vi "Main.vi"() -> ()   [LabVIEW 2021]
doc: "This vi acts as an user interface to display acquire data and save data when required. User can ineract with the panel to choose file (CSV or TDMS) and data display type(chart or graph). It also allow user to select channel index and define channel name, scale and offset. It then can let user choose a moment to start recording either on defined time length or user choice."
uses:
  Control/Data Display Choice Enum.ctl
  Control/File Choice Enum.ctl
  Control/User Interface Reference Cluster.ctl
  Control/Data Display Manager Enum.ctl
  Control/Volt Chl.ctl
  Control/File Manager Enum.ctl
  Control/Command and Data Cluster.ctl
  Control/DAQ Manager Enum.ctl
  <extravilib>/ChannelInstances/Stream-a[.](wfm(dbl))/Read With Abort.vi
  <extravilib>/ChannelInstances/Stream-a[.](wfm(dbl))/Write With Abort.vi
  <extravilib>/ChannelInstances/Stream-a[.](wfm(dbl))/EndpointRead.vi
  <extravilib>/ChannelInstances/Stream-a[.](wfm(dbl))/Endpoint.vi
  <extravilib>/ChannelInstances/Stream-a[.](wfm(dbl))/Instantiate.vi
  <extravilib>/ChannelInstances/Event Messenger-t'Command and Data Cluster.ctl'/Instantiate.vi
  <extravilib>/ChannelInstances/Event Messenger-t'Command and Data Cluster.ctl'/))Channel.vi
  <extravilib>/ChannelInstances/Stream-a[.](wfm(dbl))/)Channel.vi
  <resource>/ChannelSupport/_ChannelSupport/WaitIfNeeded.vi
  <extravilib>/ChannelInstances/Event Messenger-t'Command and Data Cluster.ctl'.lvlib
  <extravilib>/ChannelInstances/Stream-a[.](wfm(dbl)).lvlib
panel:
  out "Error":errorcluster
  out "Overall Raw \nVoltage Mean":dbl[](array[numeric])
  out "Raw Voltage Mean \nper Second":dbl[](array[numeric])
  out "Recording":bool
  in  "File Choice":T1=enum."CSV File"
  in  "DD Choice":T2 caption="Data Display Choice"
  out "File Path":path
  in  "Choice Ok":bool
  in  "File Name":string
  in  "Exit":bool
  in  "Use Re Time":bool caption="Use Record Time"
  in  "Re Time":dbl=10.0 caption="Record Time (s)"
  in  "Device Name":tag
  in  "Sample Rate":i32=100 caption="Sample Rate (S/s)"
  in  "Init Button":bool
  in  "Record":bool
  in  "Start":bool
  in  "Stop":bool
  out "element":waveform(dbl)[](array[waveform])
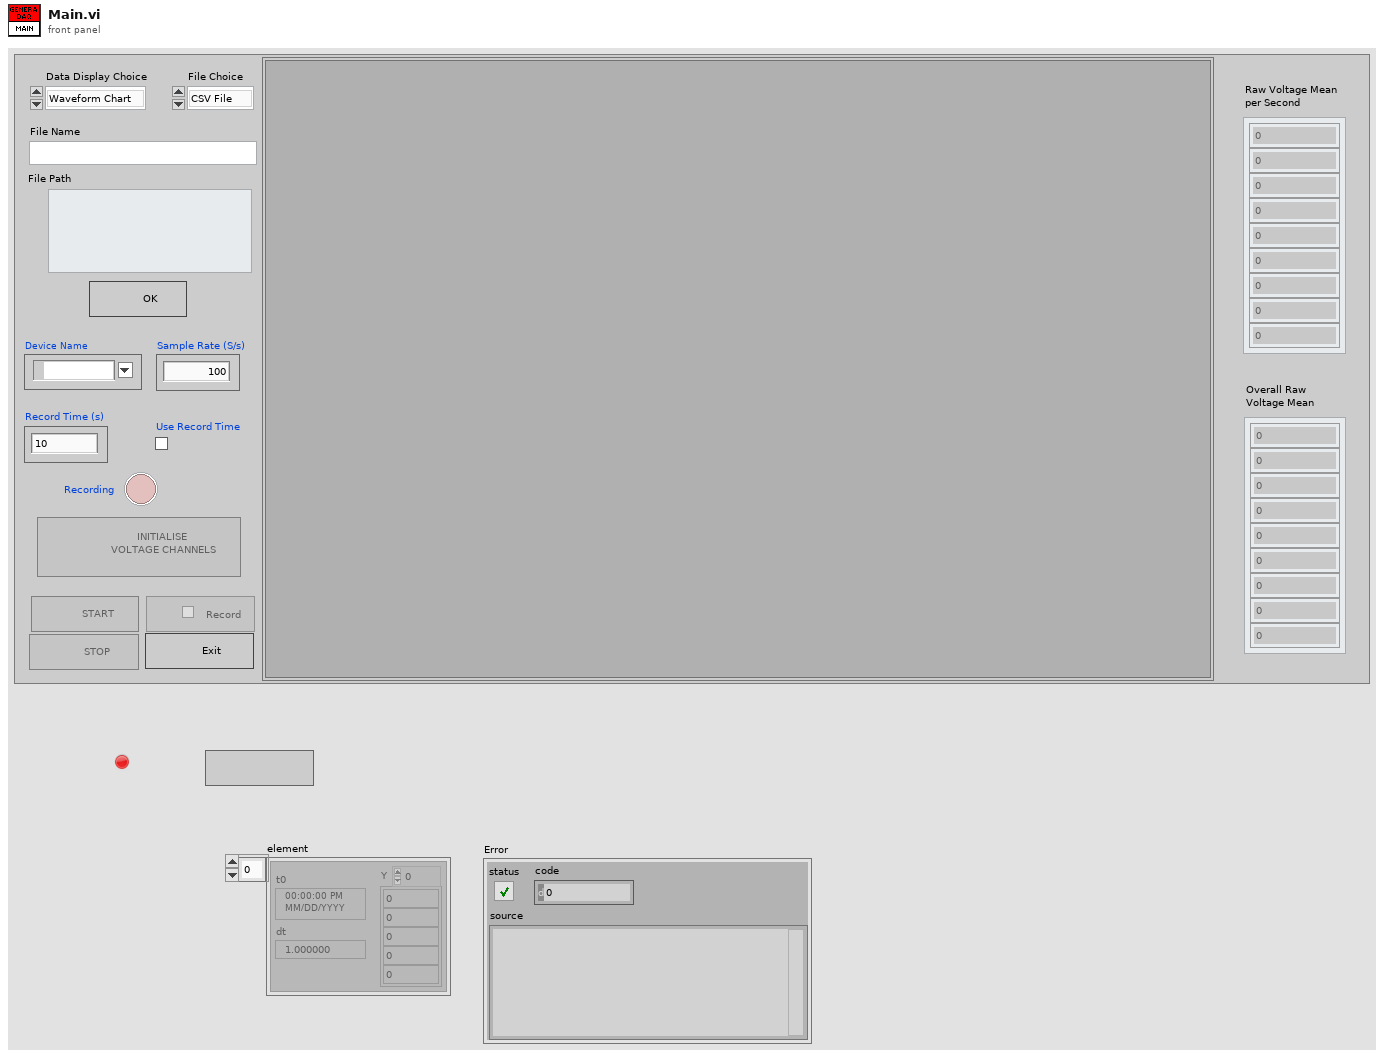
[diagram p1: front panel]
types:
  T1 = typedef "File Choice Enum.ctl" = enum16{"TDMS File", "CSV File"}
  T2 = typedef "Data Display Choice Enum.ctl" = enum16{"Waveform Chart", "Waveform Graph"}
  T3 = typedef "User Interface Reference Cluster.ctl" = cluster{"Choice Ok":refnum<vi>, "Init Button":refnum<vi>, "Start":refnum<vi>, "Record":refnum<vi>, "Stop":refnum<vi>, "Exit":refnum<vi>, "File Choice":refnum<vi>, "DD Choice":refnum<vi>}
  T4 = typedef "Command and Data Cluster.ctl" = cluster{"Command":string, "Data":variant}
  T5 = typedef "Event Messenger-t'Command and Data Cluster.ctl'.lvlib/))Channel.ctl" = refnum<queue>
  T6 = typedef "DAQ Manager Enum.ctl" = enum16{"Config", "Start", "Read", "Stop"}
  T7 = typedef "Volt Chl.ctl" = cluster{"Index":i32[], "Chl Name":string[], "Scale":dbl[], "Offset":dbl[], "Sample Rate":i32, "Device Name":tag, "Channel":tag}
  T8 = typedef "Stream-a[.](wfm(dbl)).lvlib/)Channel.ctl" = refnum<queue>
  T9 = typedef "Data Display Manager Enum.ctl" = enum16{"Display Choice", "Config Data", "Volt Data"}
  T10 = typedef "File Manager Enum.ctl" = enum16{"Create File", "Config Data", "Volt Data", "Set Time", "Close File"}
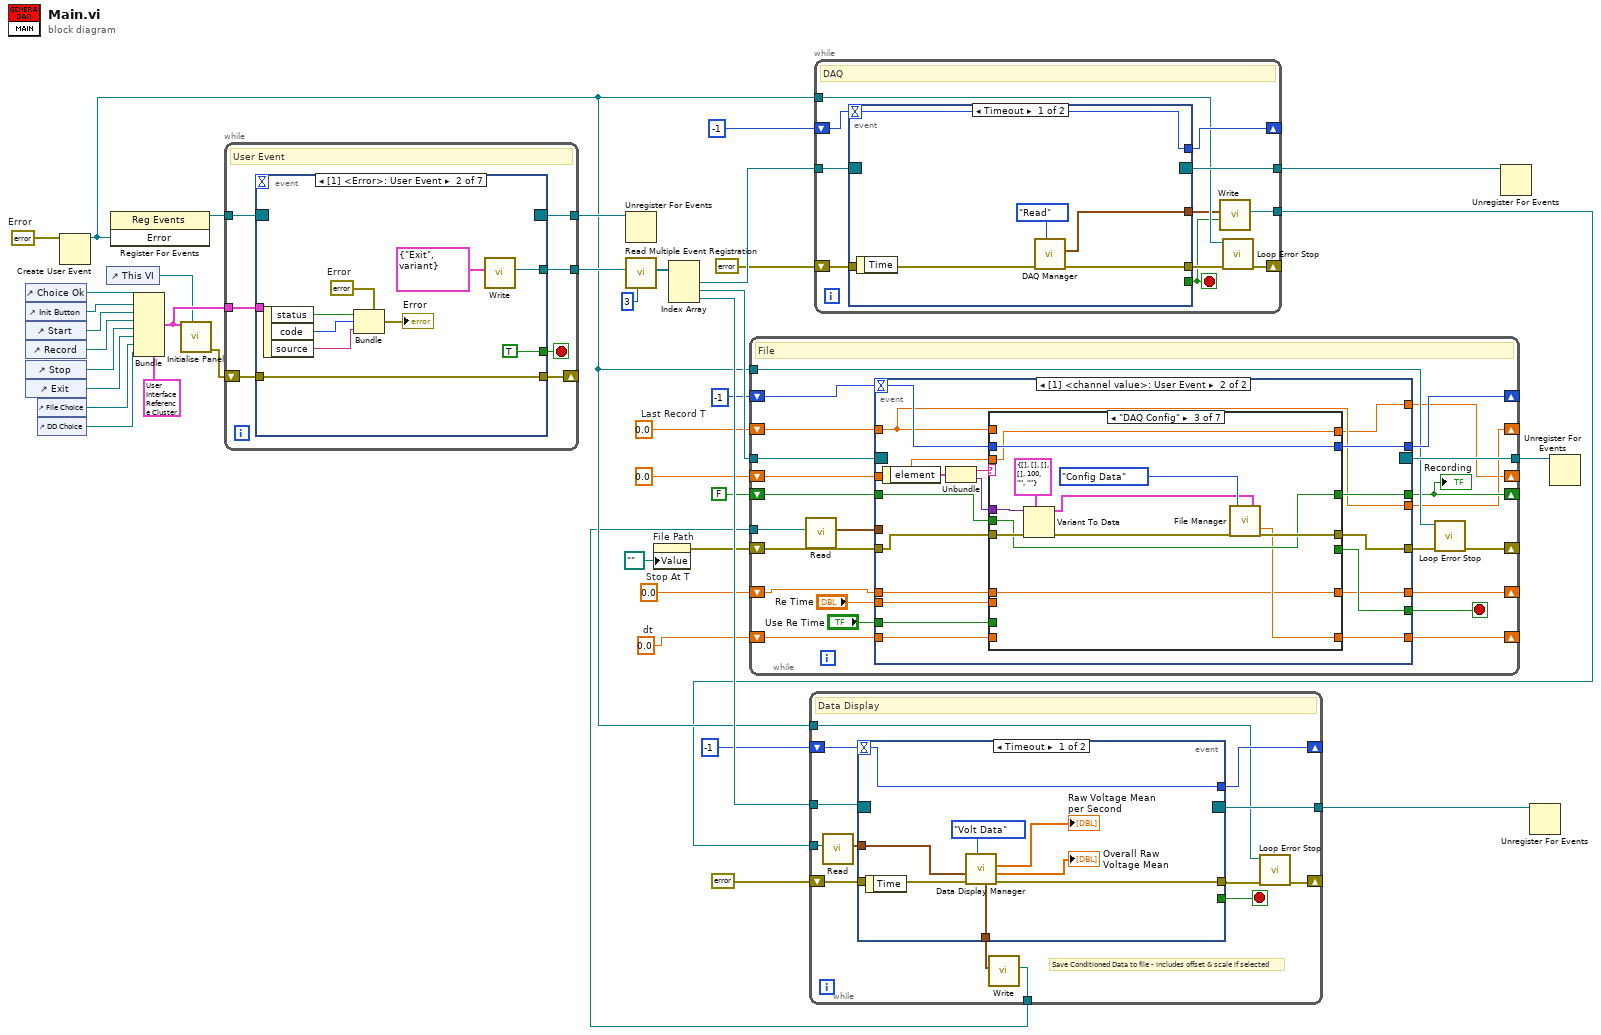
[diagram p0: block diagram]
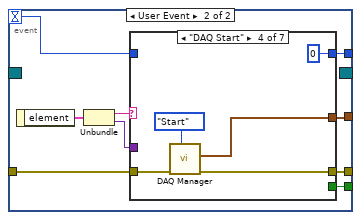
[diagram p2: hidden frame]
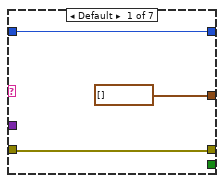
[diagram p3: hidden frame]
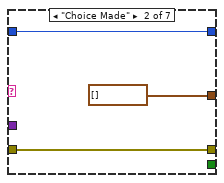
[diagram p4: hidden frame]
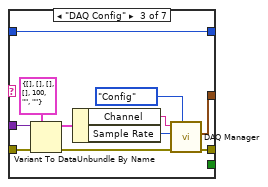
[diagram p5: hidden frame]
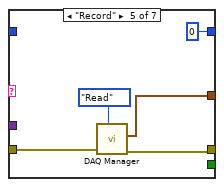
[diagram p6: hidden frame]
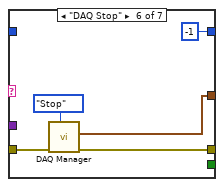
[diagram p7: hidden frame]
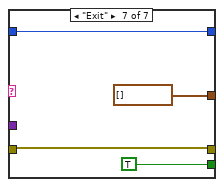
[diagram p8: hidden frame]
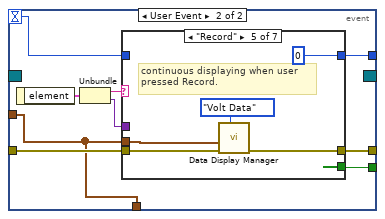
[diagram p9: hidden frame]
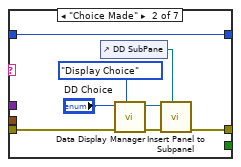
[diagram p11: hidden frame]
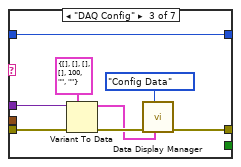
[diagram p12: hidden frame]
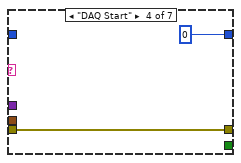
[diagram p13: hidden frame]
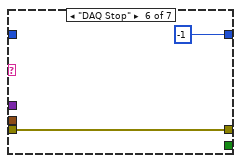
[diagram p14: hidden frame]
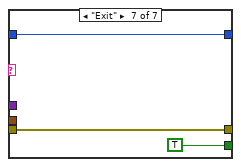
[diagram p15: hidden frame]
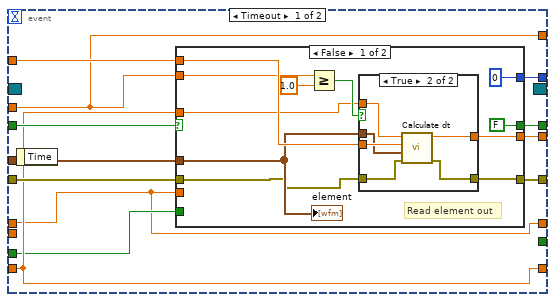
[diagram p16: hidden frame]
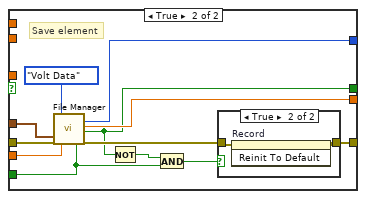
[diagram p18: hidden frame]
diagram:
  w3 = 0.0  # Stop At T
  w5 = 0.0  # dt
  w6 = 0.0  # Last Record T
  w10 = errorcluster {"status"=FALSE, "code"=0, "source"=""}  # Error
  n1 = control-ref of="Choice Ok"() -> (w27:refnum<vi>)
  n2 = control-ref of="Init Button"() -> (w26:refnum<vi>)
  n3 = control-ref of="Start"() -> (w25:refnum<vi>)
  n4 = control-ref of="Record"() -> (w24:refnum<vi>)
  n5 = control-ref of="Stop"() -> (w23:refnum<vi>)
  n6 = control-ref of="Exit"() -> (w22:refnum<vi>)
  n7 = control-ref of="File Choice"() -> (w21:refnum<vi>)
  n8 = control-ref of="DD Choice"() -> (w20:refnum<vi>)
  n9 = Create User Event(user event datatype=w10) -> (user event=w12:refnum<user-event>)  [unwired: 1 in, 1 out]
  n10 = control-ref of="This VI"() -> (w11:refnum<vi>)
  n11 = register-events(w12) -> (reference out=w14:refnum<event-registration>)  [unwired: 2 in, 1 out]
  n12 = Bundle(cluster=T3 {"Choice Ok"=refnum, "Init Button"=refnum, "Start"=refnum, "Record"=refnum, "Stop"=refnum, "Exit"=refnum, "File Choice"=refnum, "DD Choice"=refnum} ("output cluster"), "Choice Ok"=w27, "Init Button"=w26, "Start"=w25, "Record"=w24, "Stop"=w23, "Exit"=w22, "File Choice"=w21, "DD Choice"=w20) -> (w17:T3)
  n13 = call "Initialise Panel.vi"("This VI"=w11, "UI Ref"=w17) -> ("error out"=w18:errorcluster)  [unwired: 9 in]
  n14 = while {
    tunnel: [w45] -> w33
    tunnel: w17 -> [w44]
    tunnel: w14 -> [w43]
    tunnel: [w42] -> w13
    shift-right: [w40] -> _
    shift-left: w18 -> [w41]
    stop <- w46 stop-if-true
    # "User Event"
    n15 = event shown="[1] <Error>: User Event" {
      selector: w43 -> [_ _ _ _ _ _ _]
      dyn-events: [_ _ _ _ _ _ _] -> w42
      timeout: _ -> [_ _ _ _ _ _ _]
      tunnel: [TRUE TRUE _ _ _ _ _] -> w46
      tunnel: [w48 w57 w73 w90 w107 w113 w130] -> w45
      tunnel: w44 -> [_ _ w72 w85 w99 _ w129]
      tunnel: w41 -> [w47 w51 w60 w75 w93 w108 w118]
      tunnel: [w47 w51 w61 w76 w94 w108 w114] -> w40
      event "Exit": Value Change {
        n16 = event-data() -> ()  [unwired: 1 in, 1 out]
        n17 = call <extravilib>:"Write.vi"("element"=T4 {"Command"="Exit", "Data"=variant} ("Cluster")) -> ("channel"=w48:T5)  [unwired: 9 in, 1 out]
      }
      event User Event {
        w56 = errorcluster {"status"=FALSE, "code"=0, "source"=""}  # Error
        n18 = event-data() -> ("status"=w55:bool, "code"=w54:i32, "source"=w53:string)  [unwired: 1 in]
        n19 = Bundle(cluster=w56, "status"=w55, "code"=w54, "source"=w53) -> (→"Error":errorcluster)
        n20 = call <extravilib>:"Write.vi"("element"=T4 {"Command"="Exit", "Data"=variant} ("Cluster")) -> ("channel"=w57:T5)  [unwired: 9 in, 1 out]
      }
      event "Choice Ok": Value Change {
        n21 = event-data() -> ()  [unwired: 1 in, 1 out]
        n22 = Unbundle By Name(w72) -> ("File Choice"=w65:refnum<vi>, "DD Choice"=w64:refnum<vi>, "Choice Ok"=w71:refnum<vi>, "Init Button"=w70:refnum<vi>)
        n23 = Build Array(w65, w64, w71) -> (w68:refnum<vi>[])
        n24 = Build Array(w70) -> (w66:refnum<vi>[])
        n25 = call "Enable UI.vi"("Enable?"=FALSE, "output cluster"=w68) -> ("error out"=w63:errorcluster)  [unwired: 9 in]
        n26 = call "Enable UI.vi"("Enable?"=TRUE, "output cluster"=w66) -> ("error out"=w62:errorcluster)  [unwired: 9 in]
        n27 = call <extravilib>:"Write.vi"("element"=T4 {"Command"="Choice Made", "Data"=variant} ("Cluster")) -> ("channel"=w73:T5)  [unwired: 9 in, 1 out]
        n28 = Merge Errors(w63, w62, w60) -> (w61:errorcluster)
      }
      event "Init Button": Value Change {
        n29 = event-data() -> ()  [unwired: 1 in, 1 out]
        n30 = Unbundle By Name(w85) -> ("Init Button"=w80:refnum<vi>, "Start"=w79:refnum<vi>)
        n31 = Build Array(w80) -> (w84:refnum<vi>[])
        n32 = Build Array(w79) -> (w83:refnum<vi>[])
        n33 = call "DAQ Channel Dlg_V0.vi"("DAQ Sample Rate (S/s)"="Sample Rate", "Device Name"="Device Name") -> ("Chl Infor"=w86:variant)  [unwired: 9 in]
        n34 = call "Enable UI.vi"("Enable?"=FALSE, "output cluster"=w84) -> ("error out"=w77:errorcluster)  [unwired: 9 in]
        n35 = call "Enable UI.vi"("Enable?"=TRUE, "output cluster"=w83) -> ("error out"=w78:errorcluster)  [unwired: 9 in]
        n36 = Bundle(cluster=T4 {"Command"="DAQ Config", "Data"=variant} ("Cluster"), "Command"="DAQ Config" ("element"), "Data"=w86) -> (w88:T4)
        n37 = Merge Errors(w77, w78, w75) -> (w76:errorcluster)
        n38 = call <extravilib>:"Write.vi"("element"=w88) -> ("channel"=w90:T5)  [unwired: 9 in, 1 out]
      }
      event "Start": Value Change {
        n39 = event-data() -> ()  [unwired: 1 in, 1 out]
        n40 = Unbundle By Name(w99) -> ("Exit"=w97:refnum<vi>, "Start"=w101:refnum<vi>, "Record"=w100:refnum<vi>, "Stop"=w98:refnum<vi>)
        n41 = Build Array(w97, w101) -> (w105:refnum<vi>[])
        n42 = Build Array(w100, w98) -> (w104:refnum<vi>[])
        n43 = call "Enable UI.vi"("Enable?"=FALSE, "output cluster"=w105) -> ("error out"=w96:errorcluster)  [unwired: 9 in]
        n44 = call "Enable UI.vi"("Enable?"=TRUE, "output cluster"=w104) -> ("error out"=w95:errorcluster)  [unwired: 9 in]
        n45 = call <extravilib>:"Write.vi"("element"=T4 {"Command"="DAQ Start", "Data"=variant} ("Cluster")) -> ("channel"=w107:T5)  [unwired: 9 in, 1 out]
        n46 = Merge Errors(w96, w95, w93) -> (w94:errorcluster)
      }
      event "Record": Value Change {
        n47 = event-data() -> ()  [unwired: 1 in, 1 out]
        n48 = To Variant(anything="Record") -> (Variant=w110:variant)
        n49 = Bundle(cluster=T4 {"Command"="Record", "Data"=variant} ("Cluster"), "Data"=w110) -> (w109:T4)  [unwired: 1 in]
        n50 = call <extravilib>:"Write.vi"("element"=w109) -> ("channel"=w113:T5)  [unwired: 9 in, 1 out]
      }
      event "Stop": Value Change {
        n51 = event-data() -> ()  [unwired: 1 in, 1 out]
        n52 = Unbundle By Name(w129) -> ("Choice Ok"=w125:refnum<vi>, "File Choice"=w126:refnum<vi>, "DD Choice"=w127:refnum<vi>, "Exit"=w123:refnum<vi>, "Record"=w122:refnum<vi>, "Stop"=w119:refnum<vi>)
        n53 = invoke on="Record" class="Bool (strict)" method="Reinit To Default"(error in=w118) -> (error out=w115:errorcluster)  [unwired: 2 in, 2 out]
        n54 = Build Array(w125, w126, w127, w123) -> (w124:refnum<vi>[])
        n55 = Build Array(w122, w119) -> (w120:refnum<vi>[])
        n56 = call "Enable UI.vi"("Enable?"=TRUE, "output cluster"=w124) -> ("error out"=w117:errorcluster)  [unwired: 9 in]
        n57 = call "Enable UI.vi"("Enable?"=FALSE, "output cluster"=w120) -> ("error out"=w116:errorcluster)  [unwired: 9 in]
        n58 = call <extravilib>:"Write.vi"("element"=T4 {"Command"="DAQ Stop", "Data"=variant} ("Cluster")) -> ("channel"=w130:T5)  [unwired: 9 in, 1 out]
        n59 = Merge Errors(w117, w116, w115) -> (w114:errorcluster)
      }
    }
  }
  n60 = Unregister For Events(event registration refnum=w13) -> ()  [unwired: 1 in, 1 out]
  n61 = call <extravilib>:"Read Multiple Event Registration.vi"("number of event structures"=u16 3, "channel"=w33) -> ("event registration refnums"=w31:refnum<event-registration>[])  [unwired: 9 in]
  n62 = property on="File Path" class="Path"("Value"=path "" ("File Path")) -> (error out=w15:errorcluster)  [unwired: 2 in, 1 out]
  n63 = Index Array(array=w31) -> (element #1=w37:refnum<event-registration>, element #2=w38:refnum<event-registration>, element #3=w36:refnum<event-registration>)  [unwired: 3 in]
  n64 = while {
    tunnel: w37 -> [w142]
    tunnel: [w141] -> w34
    shift-right: [w139] -> _
    shift-left: -1 -> [w140]
    tunnel: [w134] -> w1
    shift-right: [w136] -> _
    shift-left: errorcluster {"status"=FALSE, "code"=0, "source"=""} ("error constant") -> [w138]
    tunnel: w12 -> [w137]
    stop <- w132 stop-if-true
    # "DAQ"
    n65 = event shown="[0] Timeout" {
      selector: w142 -> [_ _]
      dyn-events: [_ _] -> w141
      timeout: w140 -> [w147 w151]
      tunnel: [w146 w156] -> w135
      tunnel: [_ w155] -> w132
      tunnel: [w147 w150] -> w139
      tunnel: w138 -> [w144 w149]
      tunnel: [w143 w148] -> w133
      event Timeout {
        n66 = event-data() -> ()  [unwired: 1 in, 1 out]
        n67 = call "DAQ Manager.vi"("Enum"=DAQ_Manager_Enum."Read", "error in"=w144) -> ("error out"=w146:errorcluster, "data"=w143:waveform(dbl)[])  [unwired: 8 in]
      }
      event User Event {
        n68 = event-data() -> ("element"=w154:T4)  [unwired: 1 in]
        n69 = Unbundle(w154) -> ("Command"=w153:string, "Data"=w152:variant)
        n70 = case shown="\"DAQ Start\"" w153 {
          tunnel: [w158 w161 w166 w177 w179 w186 w190] -> w156
          tunnel: [_ _ _ _ _ _ TRUE] -> w155
          tunnel: w152 -> [_ _ w173 _ _ _ _]
          tunnel: w151 -> [w159 w162 w165 _ _ _ w192]
          tunnel: [w159 w162 w165 0 0 -1 w192] -> w150
          tunnel: w149 -> [w158 w161 w164 w175 w180 w185 w190]
          tunnel: [waveform(dbl)[] [] ("element") waveform(dbl)[] [] ("element") w163 w174 w181 w184 waveform(dbl)[] [] ("element")] -> w148
          frame Default {
          }
          frame "Choice Made" {
          }
          frame "DAQ Config" {
            n71 = Variant To Data(error in=w164, type=T7 {"Index"=[], "Chl Name"=[], "Scale"=[], "Offset"=[], "Sample Rate"=100, "Device Name"="", "Channel"=""} ("Volt Channel"), Variant=w173) -> (data=w171:T7, error out=w168:errorcluster)
            n72 = Unbundle By Name(w171) -> ("Channel"=w170:tag, "Sample Rate"=w169:i32)
            n73 = call "DAQ Manager.vi"("Enum"=DAQ_Manager_Enum."Config", "error in"=w168, "Sample Rate"=w169, "Chl"=w170) -> ("error out"=w166:errorcluster, "data"=w163:waveform(dbl)[])  [unwired: 6 in]
          }
          frame "DAQ Start" {
            n74 = call "DAQ Manager.vi"("Enum"=DAQ_Manager_Enum."Start", "error in"=w175) -> ("error out"=w177:errorcluster, "data"=w174:waveform(dbl)[])  [unwired: 8 in]
          }
          frame "Record" {
            n75 = call "DAQ Manager.vi"("Enum"=DAQ_Manager_Enum."Read", "error in"=w180) -> ("error out"=w179:errorcluster, "data"=w181:waveform(dbl)[])  [unwired: 8 in]
          }
          frame "DAQ Stop" {
            n76 = call "DAQ Manager.vi"("Enum"=DAQ_Manager_Enum."Stop", "error in"=w185) -> ("error out"=w186:errorcluster, "data"=w184:waveform(dbl)[])  [unwired: 8 in]
          }
          frame "Exit" {
          }
        }
      }
    }
    n77 = call <extravilib>:"Write.vi"("last element? (F)"=w132, "element"=w133) -> ("channel"=w134:T8)  [unwired: 7 in, 2 out]
    n78 = call "Loop Error Stop.vi"("error in"=w135, "user event"=w137) -> ("error out"=w136:errorcluster)  [unwired: 9 in]
  }
  n79 = while {
    tunnel: w36 -> [w205]
    tunnel: [w204] -> w35
    shift-right: [w201] -> _
    shift-left: -1 -> [w202]
    tunnel: w1 -> [w200]
    shift-right: [w196] -> _
    shift-left: errorcluster {"status"=FALSE, "code"=0, "source"=""} ("error constant") -> [w198]
    tunnel: w12 -> [w195]
    tunnel: [w193] -> w2
    stop <- w203 stop-if-true
    # "Save Conditioned Data to file - includes offset & scale if selected"
    # "Data Display"
    n80 = call <extravilib>:"Read.vi"("channel"=w200) -> ("element"=w199:waveform(dbl)[])  [unwired: 6 in, 4 out]
    n81 = event shown="[0] Timeout" {
      selector: w205 -> [_ _]
      dyn-events: [_ _] -> w204
      timeout: w202 -> [w209 w217]
      tunnel: [_ w222] -> w203
      tunnel: [w213 w221] -> w197
      tunnel: [w209 w216] -> w201
      tunnel: w199 -> [w211 w214]
      tunnel: w198 -> [w210 w215]
      tunnel: [w206 w214] -> w194
      event Timeout {
        n82 = event-data() -> ()  [unwired: 1 in, 1 out]
        n83 = call "Data Display Manager.vi"("Enum"=Data_Display_Manager_Enum."Volt Data", "error in"=w210, "Raw Data"=w211) -> ("error out"=w213:errorcluster, "Overall Mean"=→"Overall Raw \nVoltage Mean":dbl[], "Mean per Second"=→"Raw Voltage Mean \nper Second":dbl[], "Conditioned Data Out"=w206:waveform(dbl)[])  [unwired: 4 in, 1 out]
      }
      event User Event {
        n84 = event-data() -> ("element"=w220:T4)  [unwired: 1 in]
        n85 = Unbundle(w220) -> ("Command"=w219:string, "Data"=w218:variant)
        n86 = case shown="\"Record\"" w219 {
          tunnel: [_ _ _ _ _ _ TRUE] -> w222
          tunnel: [w223 w227 w238 w241 w243 w248 w250] -> w221
          tunnel: w218 -> [_ _ w236 _ _ _ _]
          tunnel: w217 -> [w224 w226 w240 _ _ _ w251]
          tunnel: [w224 w226 w240 0 0 -1 w251] -> w216
          tunnel: w215 -> [w223 w225 w233 w241 w244 w248 w250]
          tunnel: w214 -> [_ _ _ _ w245 _ _]
          frame Default {
          }
          frame "Choice Made" {
            n87 = control-ref of="DD SubPane"() -> (w230:refnum<vi>)
            n88 = call "Data Display Manager.vi"("Enum"=Data_Display_Manager_Enum."Display Choice", "error in"=w225, "Data Display Choice"="DD Choice") -> ("error out"=w228:errorcluster, "VI Ref"=w229:refnum<vi>)  [unwired: 4 in, 3 out]
            n89 = call "Insert Panel to Subpanel.vi"("SubPanel in"=w230, "error in"=w228, "VI Ref"=w229) -> ("error out"=w227:errorcluster)  [unwired: 8 in]
          }
          frame "DAQ Config" {
            n90 = Variant To Data(error in=w233, type=T7 {"Index"=[], "Chl Name"=[], "Scale"=[], "Offset"=[], "Sample Rate"=100, "Device Name"="", "Channel"=""} ("Volt Channel"), Variant=w236) -> (data=w234:T7, error out=w235:errorcluster)
            n91 = call "Data Display Manager.vi"("Volt Channel"=w234, "Enum"=Data_Display_Manager_Enum."Config Data", "error in"=w235) -> ("error out"=w238:errorcluster)  [unwired: 4 in, 4 out]
          }
          frame "DAQ Start" {
          }
          frame "Record" {
            # "continuous displaying when user\npressed Record."
            n92 = call "Data Display Manager.vi"("Enum"=Data_Display_Manager_Enum."Volt Data", "error in"=w244, "Raw Data"=w245) -> ("error out"=w243:errorcluster)  [unwired: 4 in, 4 out]
          }
          frame "DAQ Stop" {
          }
          frame "Exit" {
          }
        }
      }
    }
    n93 = call <extravilib>:"Write.vi"("element"=w194) -> ("channel"=w193:T8)  [unwired: 8 in, 2 out]
    n94 = call "Loop Error Stop.vi"("error in"=w197, "user event"=w195) -> ("error out"=w196:errorcluster)  [unwired: 9 in]
  }
  n95 = while {
    tunnel: w38 -> [w275]
    tunnel: [w274] -> w39
    tunnel: w2 -> [w253]
    shift-right: [w266] -> _
    shift-left: w15 -> [w272]
    shift-right: [w269] -> _
    shift-left: -1 -> [w270]
    shift-right: [w264] -> _
    shift-left: FALSE ("Recording") -> [w268]
    tunnel: w12 -> [w265]
    shift-right: [w262] -> _
    shift-left: w6 -> [w263]
    shift-right: [w260] -> _
    shift-left: w5 -> [w261]
    shift-right: [w258] -> _
    shift-left: 0.0 -> [w259]
    shift-right: [w254] -> _
    shift-left: w3 -> [w255]
    stop <- w273 stop-if-true
    # "File"
    n96 = call <extravilib>:"Read.vi"("channel"=w253) -> ("element"=w271:waveform(dbl)[])  [unwired: 6 in, 4 out]
    n97 = event shown="[1] <channel value>: User Event" {
      selector: w275 -> [_ _]
      dyn-events: [_ _] -> w274
      timeout: w270 -> [_ w335]
      tunnel: [w286 w340] -> w267
      tunnel: [_ w339] -> w273
      tunnel: w272 -> [w287 w326]
      tunnel: w271 -> [w285 _]
      tunnel: [w283 w334] -> w269
      tunnel: [w282 w333] -> w264
      tunnel: w268 -> [w284 w332]
      tunnel: w263 -> [w280 w331]
      tunnel: [w281 w331] -> w262
      tunnel: w261 -> [w278 w329]
      tunnel: [w278 w330] -> w260
      tunnel: w259 -> [w279 w327]
      tunnel: [w279 w328] -> w258
      tunnel: "Re Time" -> [_ w324]
      tunnel: "Use Re Time" -> [w277 w325]
      tunnel: w255 -> [w276 w323]
      tunnel: [w276 w322] -> w254
      event Timeout {
        n98 = event-data() -> ()  [unwired: 1 in, 1 out]
        n99 = case shown="False" w284 {
          tunnel: w287 -> [w293 w318]
          tunnel: [w292 w313] -> w286
          tunnel: w285 -> [w294 w316]
          tunnel: [0 ("timeout") w315] -> w283
          tunnel: w277 -> [_ w310]
          tunnel: [FALSE ("Recording") w307] -> w282
          tunnel: [w295 w312] -> w281
          tunnel: w280 -> [w296 _]
          tunnel: w279 -> [w291 _]
          tunnel: w278 -> [w288 _]
          tunnel: w276 -> [_ w311]
          frame False {
            # "Read element out"
            n100 = Greater Or Equal?(x=w291, y=1.0) -> (x >= y?=w289:bool)
            n101 = case shown="True" w289 {
              tunnel: w296 -> [w300 w306]
              tunnel: [w300 w305] -> w295
              tunnel: w294 -> [_ w304]
              tunnel: w293 -> [w299 w303]
              tunnel: [w299 w302] -> w292
              tunnel: w288 -> [_ w301]
              frame False {
              }
              frame True {
                n102 = call "Calculate dt.vi"("error in"=w303, "Voltage in"=w304, "t_start in"=w306, "dt"=w301) -> ("error out"=w302:errorcluster, "t_start out"=w305:dbl)  [unwired: 6 in]
              }
            }
            "element" <- w294
          }
          frame True {
            # "Save element"
            n103 = call "File Manager.vi"("Voltage"=w316, "error in"=w318, "Enum"=File_Manager_Enum."Volt Data", "Record Time (s)"=w311, "Use Record Time"=w310) -> ("timeout"=w315:i32, "ET out"=w312:dbl, "Recording"=w307:bool, "error out"=w314:errorcluster)  [unwired: 9 in, 2 out]
            n104 = Not(x=w307) -> (.not. x?=w308:bool)
            n105 = And(x=w308, y=w310) -> (x .and. y?=w309:bool)
            n106 = case shown="True" w309 {
              tunnel: w314 -> [w319 w321]
              tunnel: [w319 w320] -> w313
              frame False {
              }
              frame True {
                n107 = invoke on="Record" class="Bool (strict)" method="Reinit To Default"(error in=w321) -> (error out=w320:errorcluster)  [unwired: 2 in, 2 out]
              }
            }
          }
        }
      }
      event User Event {
        n108 = event-data() -> ("element"=w338:T4)  [unwired: 1 in]
        n109 = Unbundle(w338) -> ("Command"=w337:string, "Data"=w336:variant)
        n110 = case shown="\"DAQ Config\"" w337 {
          tunnel: [w345 w355 w368 w375 w386 w410 w419] -> w340
          tunnel: [_ _ _ _ _ _ TRUE] -> w339
          tunnel: w336 -> [_ _ w367 _ w390 _ _]
          tunnel: w326 -> [w345 w351 w363 w375 w389 w411 w419]
          tunnel: w335 -> [w346 w352 w362 _ _ _ w421]
          tunnel: [w346 w352 w362 0 0 -1 w421] -> w334
          tunnel: [w344 w350 w361 w373 w378 FALSE w418] -> w333
          tunnel: w332 -> [w344 w350 w361 w373 _ _ w418]
          tunnel: w331 -> [_ _ _ _ w381 _ _]
          tunnel: [w343 w349 w360 w372 w385 w409 w417] -> w330
          tunnel: w329 -> [w343 w349 _ w372 w385 w409 w417]
          tunnel: [w342 w348 w359 w371 1.0 w408 w416] -> w328
          tunnel: w327 -> [w342 w348 w359 w371 _ w408 w416]
          tunnel: w325 -> [_ _ _ _ w383 _ _]
          tunnel: w324 -> [_ _ _ _ w382 _ _]
          tunnel: w323 -> [w341 w347 w358 w370 w379 w407 w415]
          tunnel: [w341 w347 w358 w370 w380 w407 w415] -> w322
          frame Default {
          }
          frame "Choice Made" {
            n111 = call "File Manager.vi"("File Name"="File Name", "File Choice"="File Choice", "error in"=w351, "Enum"=File_Manager_Enum."Create File") -> ("File Path"=→"File Path":path, "error out"=w355:errorcluster)  [unwired: 10 in, 4 out]
          }
          frame "DAQ Config" {
            n112 = Variant To Data(error in=w363, type=T7 {"Index"=[], "Chl Name"=[], "Scale"=[], "Offset"=[], "Sample Rate"=100, "Device Name"="", "Channel"=""} ("Volt Channel"), Variant=w367) -> (data=w364:T7, error out=w365:errorcluster)
            n113 = call "File Manager.vi"("error in"=w365, "Enum"=File_Manager_Enum."Config Data", "Volt Channel"=w364) -> ("dt Out"=w360:dbl, "error out"=w368:errorcluster)  [unwired: 11 in, 4 out]
          }
          frame "DAQ Start" {
          }
          frame "Record" {
            # "output 1 to n"
            n114 = Variant To Data(error in=w389, type=TRUE, Variant=w390) -> (data=w378:bool, error out=w377:errorcluster)
            n115 = case shown="True" w378 {
              tunnel: w383 -> [_ w400]
              tunnel: w382 -> [_ w399]
              tunnel: w381 -> [_ w398]
              tunnel: [w392 w397] -> w380
              tunnel: w379 -> [w392 w396]
              tunnel: w377 -> [w393 w395]
              tunnel: [w393 w394] -> w376
              frame False {
              }
              frame True {
                n116 = case shown="True" w400 {
                  tunnel: w399 -> [_ w404]
                  tunnel: w398 -> [_ w406]
                  tunnel: [w402 w405] -> w397
                  tunnel: w396 -> [w402 _]
                  tunnel: w395 -> [w401 w403]
                  tunnel: [w401 w403] -> w394
                  frame False {
                  }
                  frame True {
                    n117 = Add(x=w406, y=w404) -> (x+y=w405:dbl)
                  }
                }
              }
            }
            n118 = call "File Manager.vi"("Existing Time"=w381, "error in"=w376, "Enum"=File_Manager_Enum."Set Time") -> ("error out"=w386:errorcluster)  [unwired: 11 in, 5 out]
          }
          frame "DAQ Stop" {
            n119 = call "File Manager.vi"("error in"=w411, "Enum"=File_Manager_Enum."Close File") -> ("error out"=w410:errorcluster)  [unwired: 12 in, 5 out]
          }
          frame "Exit" {
          }
        }
      }
    }
    "Recording" <- w264
    n120 = call "Loop Error Stop.vi"("error in"=w267, "user event"=w265) -> ("error out"=w266:errorcluster)  [unwired: 9 in]
  }
  n121 = Unregister For Events(event registration refnum=w34) -> ()  [unwired: 1 in, 1 out]
  n122 = Unregister For Events(event registration refnum=w35) -> ()  [unwired: 1 in, 1 out]
  n123 = Unregister For Events(event registration refnum=w39) -> ()  [unwired: 1 in, 1 out]
